vi "PID Gain Schedule.vi"   [LabVIEW 2020, in "NI_PID_pid.lvlib"]
doc: "Selects a set of PID gains from a gain schedule for the control of processes that require different sets of gains for different regions of operation, such as highly nonlinear processes. Use the DBL instance of this VI to implement a single control loop. Use the DBL Array instance to implement parallel multi-loop control."
uses:
  NI_PID_pid.lvlib
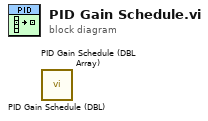
[diagram p0: block diagram]
diagram:
  n1 = call "PID Gain Schedule (DBL).vi"() -> ()  [unwired: 4 in, 2 out]
  n2 = call "PID Gain Schedule (DBL Array).vi"() -> ()  [unwired: 4 in, 2 out]
